vi "Create New Test Case.vi"(8 "error in (no error)":errorcluster) -> (0 "error out":errorcluster)   [LabVIEW 2020, in "New Test Case.lvlib"]
uses:
  New Test Case.lvlib
  <vilib>/Utility/sysdir.llb/System Directory Type.ctl
  <vilib>/Utility/error.llb/Error Cluster From Error Code.vi
  <vilib>/ErrorRing/Error Ring.xnode
panel:
  in  "Debug?":bool
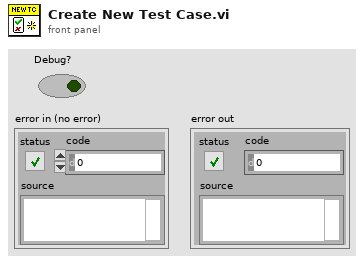
[diagram p1: front panel]
types:
  T1 = enum32{"Invalid", "Standard", "Closed", "Hidden", "Minimized", "Maximized"}
  T2 = typedef "System Directory Type.ctl" = i32
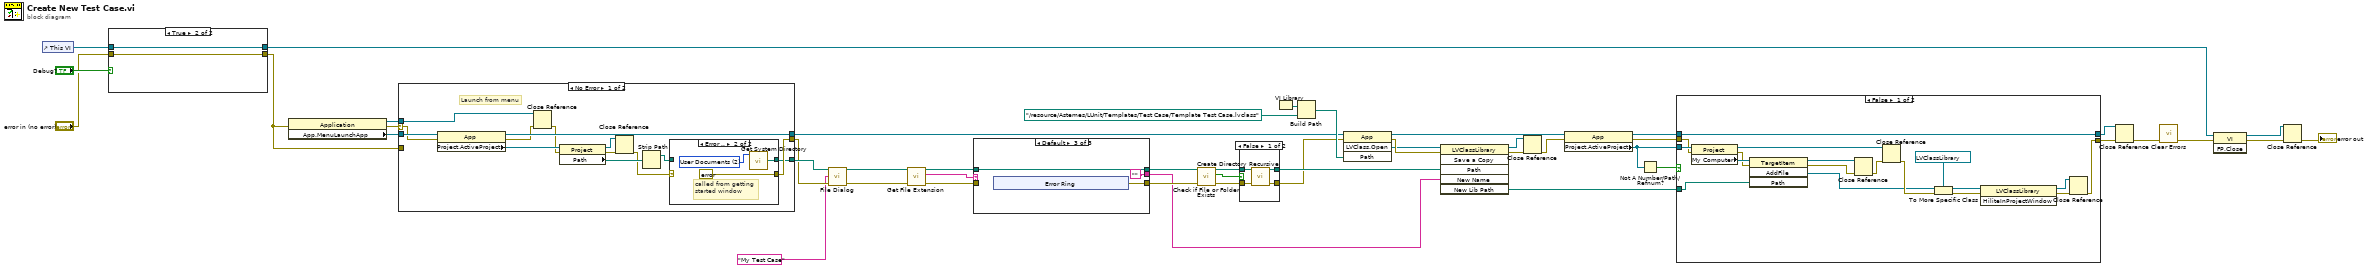
[diagram p0: block diagram]
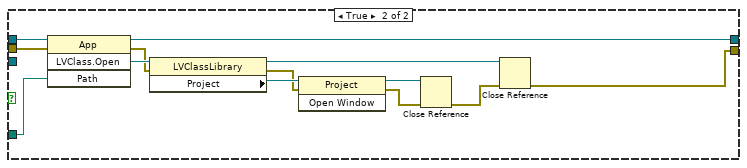
[diagram p2: hidden frame]
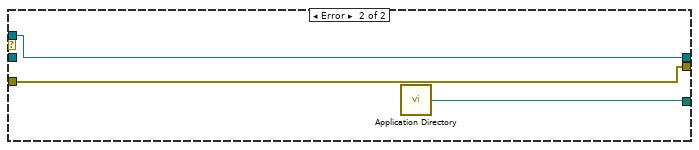
[diagram p4: hidden frame]
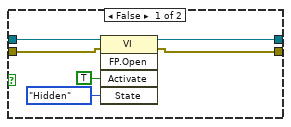
[diagram p5: hidden frame]
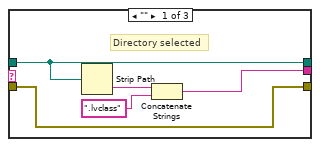
[diagram p6: hidden frame]
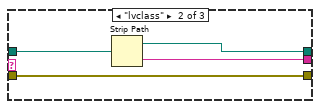
[diagram p7: hidden frame]
diagram:
  n1 = control-ref of="This VI"() -> (w17:refnum<vi>)
  n2 = case shown="True" "Debug?" {
    tunnel: w17 -> [w52 w54]
    tunnel: [w51 w54] -> w15
    tunnel: "error in (no error)" -> [w48 w53]
    tunnel: [w47 w53] -> w6
    frame False {
      n3 = invoke class="VI" method="FP.Open"(reference=w52, error in=w48, "Activate"=TRUE ("Activate?"), "State"=T1."Hidden") -> (reference out=w51:refnum<vi>, error out=w47:errorcluster)  [unwired: 1 in, 3 out]
    }
    frame True {
    }
  }
  n4 = property class="Application"(error in=w6) -> (reference out=w12:refnum<vi>, error out=w20:errorcluster, "App.MenuLaunchApp"=w46:refnum<vi>)  [unwired: 1 in]
  n5 = case shown="No Error" w20 {
    selector: w20 -> [w63 _]
    tunnel: [w66 w76] -> w8
    tunnel: w46 -> [w64 _]
    tunnel: [w57 w75] -> w4
    tunnel: w6 -> [_ w75]
    tunnel: w12 -> [w68 w76]
    tunnel: [w56 w74] -> w5
    frame No Error {
      # "Launch from menu"
      n6 = property class="App"(reference=w64, error in=w63) -> (reference out=w66:refnum<vi>, error out=w65:errorcluster, "Project.ActiveProject"=w67:refnum<vi>)
      n7 = Close Reference(reference=w68, error in (no error)=w65) -> (error out=w62:errorcluster)
      n8 = property class="Project"(reference=w67, error in=w62) -> (reference out=w60:refnum<vi>, error out=w61:errorcluster, "Path"=w59:path)
      n9 = Close Reference(reference=w60, error in (no error)=w61) -> (error out=w58:errorcluster)
      n10 = Strip Path(path=w59) -> (stripped path=w55:path)  [unwired: 1 out]
      n11 = case shown="Error .." w58 {
        selector: w58 -> [w70 _]
        tunnel: [w70 errorcluster {"status"=FALSE, "code"=0, "source"=""} ("error IO")] -> w57
        tunnel: [w69 w71] -> w56
        tunnel: w55 -> [w69 _]
        frame No Error {
        }
        frame Error {
          w72 = T2 2 items=["User Home"=0, "User Desktop"=1, "User Documents"=2, "User Application Data"=3, "User Preferences"=4, "User Temporary"=5, "Public Documents"=6, "Public Application Data"=7, "Public Preferences"=8, "Public Cache"=13, "System Core Libraries"=9, "System Installed Libraries"=10, "Application Files"=11, "Boot Volume Root"=12] ("system directory type")
          # "called from getting started window"
          n12 = call <vilib>:"Get System Directory.vi"("system directory type"=w72) -> ("system directory"=w71:path)  [unwired: 10 in]
        }
      }
    }
    frame Error {
      n13 = call <vilib>:"Application Directory.vi"() -> ("Application Directory"=w74:path)
    }
  }
  n14 = call "File Dialog"("start path"=w5, "default name"="My Test Case", "error in"=w4) -> ("selected path"=w42:path, "error out"=w3:errorcluster)  [unwired: 9 in, 2 out]
  n15 = call <vilib>:"Get File Extension.vi"("error in (no error)"=w3, "file"=w42) -> ("error out"=w45:errorcluster, "lowercase file extension"=w44:string, "dup file"=w43:path)  [unwired: 5 in, 2 out]
  n16 = case shown="Default" w44 {
    tunnel: w45 -> [w77 w82 _]
    tunnel: w43 -> [w78 w85 w86]
    tunnel: [w77 w82 w88] -> w40
    tunnel: [w79 w84 "" ("name")] -> w35
    tunnel: [w78 w83 w86] -> w41
    frame "" {
      # "Directory selected"
      n17 = Strip Path(path=w78) -> (name=w81:string)  [unwired: 1 out]
      n18 = Concatenate Strings(w81, ".lvclass" ("string")) -> (w79:string)
    }
    frame "lvclass" {
      n19 = Strip Path(path=w85) -> (stripped path=w83:path, name=w84:string)
    }
    frame Default {
      n20 = xnode "Error Ring"() -> ("error out"=w88:errorcluster)
    }
  }
  n21 = call <vilib>:"Check if File or Folder Exists.vi"("error in (no error)"=w40, "path"=w41) -> ("error out"=w39:errorcluster, "file or folder exists?"=w37:bool, "dup path"=w38:path)  [unwired: 7 in]
  n22 = case shown="False" w37 {
    tunnel: w39 -> [w96 w97]
    tunnel: w38 -> [w95 w98]
    tunnel: [w94 w98] -> w36
    tunnel: [w93 w97] -> w2
    frame False {
      n23 = call <vilib>:"Create Directory Recursive.vi"("error in (no error)"=w96, "directory"=w95) -> ("error out"=w93:errorcluster, "directory copy"=w94:path)  [unwired: 3 in, 1 out]
    }
    frame True {
    }
  }
  n24 = VI Library() -> (path=w26:path)
  n25 = Build Path(base path=w26, name or relative path=path "../resource/Astemes/LUnit/Templates/Test Case/Template Test Case.lvclass") -> (appended path=w24:path)
  n26 = invoke class="App" method="LVClass.Open"(reference=w8, error in=w2, "Path"=w24) -> (reference out=w21:refnum<vi>, error out=w34:errorcluster, "LVClass.Open"=w13:refnum<vi>)  [unwired: 1 in, 1 out]
  n27 = invoke class="LVClassLibrary" method="Save a Copy"(reference=w13, error in=w34, "Path"=w36, "New Name"=w35) -> (reference out=w22:refnum<vi>, error out=w19:errorcluster, "New Lib Path"=w30:path)  [unwired: 2 in, 3 out]
  n28 = Close Reference(reference=w22, error in (no error)=w19) -> (error out=w18:errorcluster)
  n29 = property class="App"(reference=w21, error in=w18) -> (reference out=w29:refnum<vi>, error out=w31:errorcluster, "Project.ActiveProject"=w32:refnum<vi>)
  n30 = Not A Number/Path/Refnum?(number/path/refnum=w32) -> (NaN/Path/Refnum?=w33:bool)
  n31 = case shown="False" w33 {
    tunnel: w32 -> [w116 _]
    tunnel: w31 -> [w114 w120]
    tunnel: w30 -> [w108 w118]
    tunnel: [w103 w117] -> w27
    tunnel: w29 -> [w107 w121]
    tunnel: [w107 w119] -> w28
    frame False {
      n32 = property class="Project"(reference=w116, error in=w114) -> (reference out=w110:refnum<vi>, error out=w113:errorcluster, "My Computer"=w115:refnum<vi>)
      n33 = invoke class="TargetItem" method="AddFile"(reference=w115, error in=w113, "Path"=w108) -> (reference out=w111:refnum<vi>, error out=w112:errorcluster, "AddFile"=w99:refnum<vi>)  [unwired: 1 in, 1 out]
      n34 = Close Reference(reference=w111, error in (no error)=w112) -> (error out=w109:errorcluster)
      n35 = Close Reference(reference=w110, error in (no error)=w109) -> (error out=w106:errorcluster)
      n36 = To More Specific Class(target class=refnum<vi> refnum ("reference"), reference=w99, error in=w106) -> (specific class reference=w100:refnum<vi>, error out=w102:errorcluster)
      n37 = invoke class="LVClassLibrary" method="HiliteInProjectWindow"(reference=w100, error in=w102) -> (reference out=w104:refnum<vi>, error out=w105:errorcluster)  [unwired: 1 in, 1 out]
      n38 = Close Reference(reference=w104, error in (no error)=w105) -> (error out=w103:errorcluster)
    }
    frame True {
      n39 = invoke class="App" method="LVClass.Open"(reference=w121, error in=w120, "Path"=w118) -> (reference out=w119:refnum<vi>, error out=w128:errorcluster, "LVClass.Open"=w129:refnum<vi>)  [unwired: 1 in, 1 out]
      n40 = property class="LVClassLibrary"(reference=w129, error in=w128) -> (reference out=w127:refnum<vi>, error out=w125:errorcluster, "Project"=w126:refnum<vi>)
      n41 = invoke class="Project" method="Open Window"(reference=w126, error in=w125) -> (reference out=w124:refnum<vi>, error out=w123:errorcluster)  [unwired: 1 in, 1 out]
      n42 = Close Reference(reference=w124, error in (no error)=w123) -> (error out=w122:errorcluster)
      n43 = Close Reference(reference=w127, error in (no error)=w122) -> (error out=w117:errorcluster)
    }
  }
  n44 = Close Reference(reference=w28, error in (no error)=w27) -> (error out=w23:errorcluster)
  n45 = call <vilib>:"Clear Errors.vi"("error in (no error)"=w23) -> ("error out"=w9:errorcluster)  [unwired: 5 in, 1 out]
  n46 = invoke class="VI" method="FP.Close"(reference=w15, error in=w9) -> (reference out=w11:refnum<vi>, error out=w10:errorcluster)  [unwired: 1 in, 1 out]
  n47 = Close Reference(reference=w11, error in (no error)=w10) -> (error out=→"error out":errorcluster)
